vi "HOST_SviTockovi.vi"() -> ()   [LabVIEW 2014]
uses:
  <vilib>/rvi/interface/nirviOpenFPGA/nirviOpenFPGA.xnode
  <vilib>/rvi/interface/nirviReadWriteControl/nirviReadWriteControl.xnode
  <vilib>/rvi/interface/nirviCloseFPGA/nirviCloseFPGA.xnode
  <vilib>/FPGAPlugInAG/Dynamic/niLvFpga_Close_Dynamic.vi
  NiFpgaLv.dll
  <vilib>/Utility/error.llb/Error Cluster From Error Code.vi
  <vilib>/rvi/interface/Simulation/niFpgaSimulationCallBeginRW.vi
  <vilib>/rvi/errors/niLvFpgaAdjustHostInterfaceError.vi
  FPGA Bitfiles/UpravljanjeSaSvi_FPGATarget_Untitled2_yLwRjzwkvq8.lvbitx
  Untitled 2.vi
  <vilib>/FPGAPlugInAG/sbRIO-9636/niLvFpga_Open_sbRIO-9636.vi
  <vilib>/rvi/interface/common/dynamic/niFpgaDynamicAddResources.vi
panel:
  in  "stop":bool
  in  "naprijed":bool
  in  "dir 4":bool
  in  "dir 3":bool
  in  "dir 2":bool
  in  "dir 1":bool
  in  "rezolucija koraka":i32(listbox)
  in  "step":sgl(knob) scale=0.0..300.0
  in  "pokreni":bool
  in  "ulijevo":bool
  in  "udesno":bool
  in  "nazad":bool
  in  "rotacija udesno":bool
  in  "rotacija ulijevo":bool
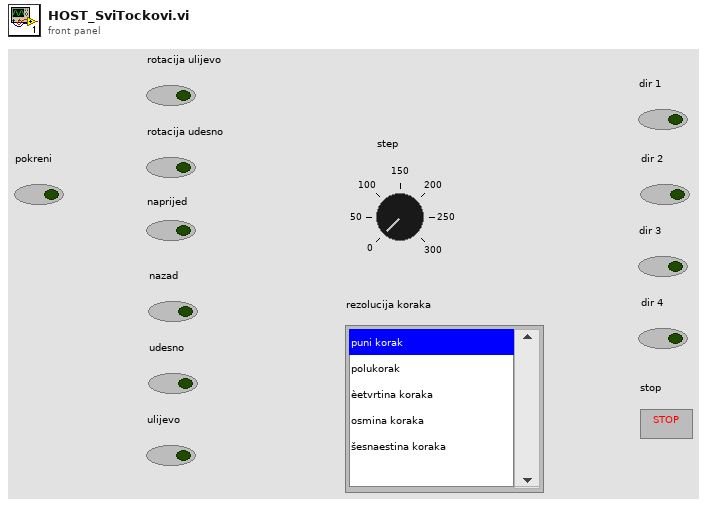
[diagram p1: front panel]
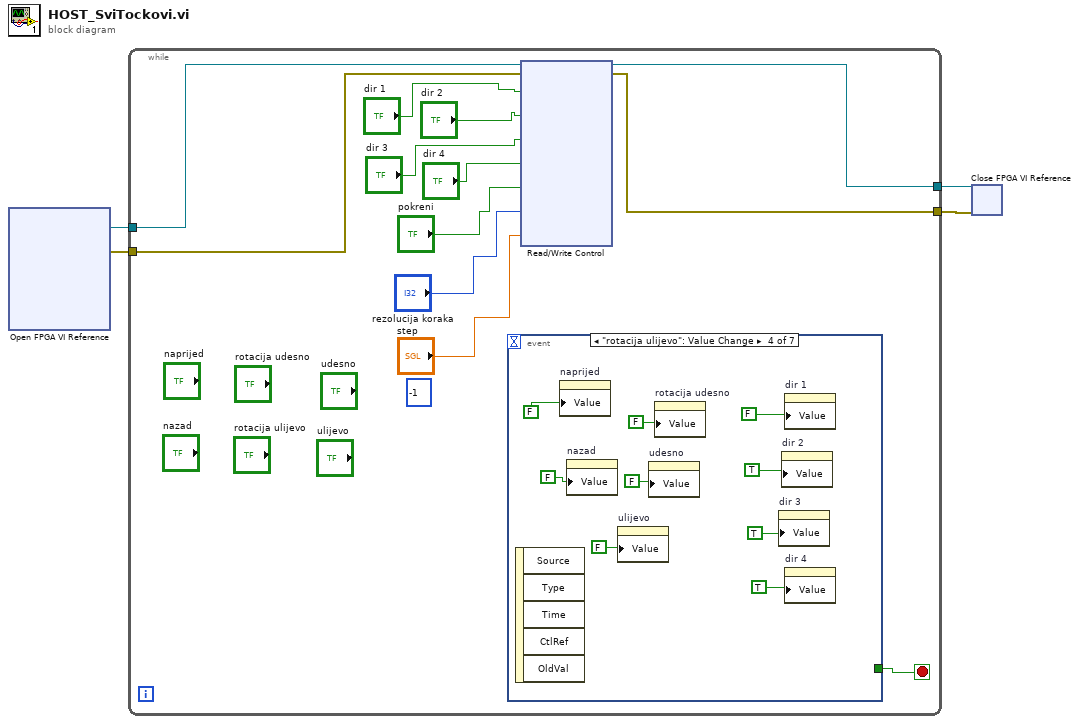
[diagram p0: block diagram]
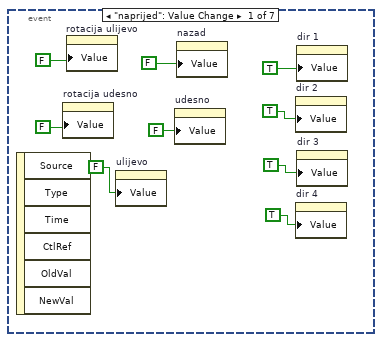
[diagram p2: hidden frame]
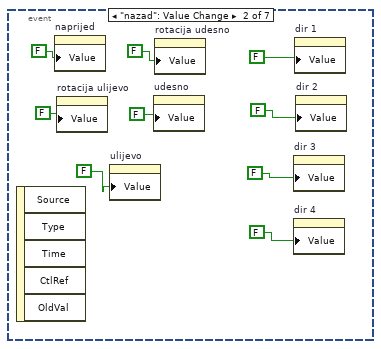
[diagram p3: hidden frame]
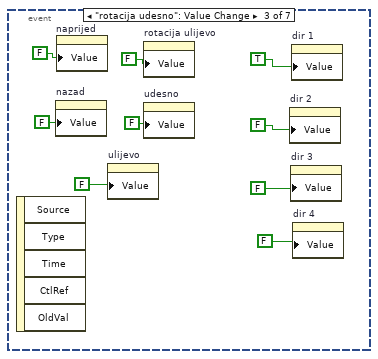
[diagram p4: hidden frame]
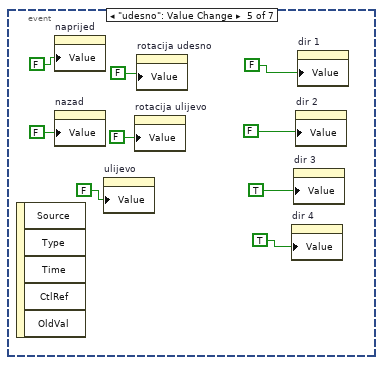
[diagram p5: hidden frame]
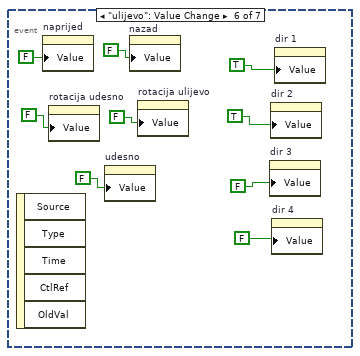
[diagram p6: hidden frame]
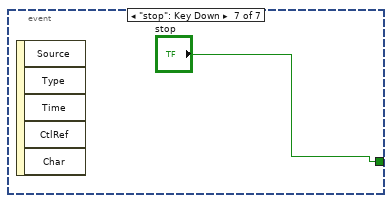
[diagram p7: hidden frame]
diagram:
  n1 = xnode "Open FPGA VI Reference"() -> ("FPGA VI Reference Out"=w3:refnum<k20>, "error out"=w4:errorcluster)  [unwired: 2 in]
  n2 = while {
    tunnel: w4 -> [w15]
    tunnel: w3 -> [w16]
    tunnel: [w14] -> w2
    tunnel: [w13] -> w1
    stop <- w5 stop-if-true
    (unwired) -1
    n3 = event shown="[3] \"rotacija ulijevo\": Value Change" {
      selector: _ -> [_ _ _ _ _ _ _]
      dyn-events: _ -> [_ _ _ _ _ _ _]
      timeout: _ -> [_ _ _ _ _ _ _]
      tunnel: [_ _ _ _ _ _ "stop"] -> w5
      event "naprijed": Value Change {
        n4 = event-data() -> ()  [unwired: 1 in, 6 out]
        n5 = property on="rotacija udesno" class="Bool (strict)"("Value"=FALSE) -> ()  [unwired: 2 in, 2 out]
        n6 = property on="rotacija ulijevo" class="Bool (strict)"("Value"=FALSE) -> ()  [unwired: 2 in, 2 out]
        n7 = property on="ulijevo" class="Bool (strict)"("Value"=FALSE) -> ()  [unwired: 2 in, 2 out]
        n8 = property on="udesno" class="Bool (strict)"("Value"=FALSE) -> ()  [unwired: 2 in, 2 out]
        n9 = property on="nazad" class="Bool (strict)"("Value"=FALSE) -> ()  [unwired: 2 in, 2 out]
        n10 = property on="dir 2" class="Bool (strict)"("Value"=TRUE) -> ()  [unwired: 2 in, 2 out]
        n11 = property on="dir 4" class="Bool (strict)"("Value"=TRUE) -> ()  [unwired: 2 in, 2 out]
        n12 = property on="dir 1" class="Bool (strict)"("Value"=TRUE) -> ()  [unwired: 2 in, 2 out]
        n13 = property on="dir 3" class="Bool (strict)"("Value"=TRUE) -> ()  [unwired: 2 in, 2 out]
      }
      event "nazad": Value Change {
        n14 = event-data() -> ()  [unwired: 1 in, 5 out]
        n15 = property on="naprijed" class="Bool (strict)"("Value"=FALSE) -> ()  [unwired: 2 in, 2 out]
        n16 = property on="rotacija ulijevo" class="Bool (strict)"("Value"=FALSE) -> ()  [unwired: 2 in, 2 out]
        n17 = property on="ulijevo" class="Bool (strict)"("Value"=FALSE) -> ()  [unwired: 2 in, 2 out]
        n18 = property on="udesno" class="Bool (strict)"("Value"=FALSE) -> ()  [unwired: 2 in, 2 out]
        n19 = property on="rotacija udesno" class="Bool (strict)"("Value"=FALSE) -> ()  [unwired: 2 in, 2 out]
        n20 = property on="dir 3" class="Bool (strict)"("Value"=FALSE) -> ()  [unwired: 2 in, 2 out]
        n21 = property on="dir 4" class="Bool (strict)"("Value"=FALSE) -> ()  [unwired: 2 in, 2 out]
        n22 = property on="dir 1" class="Bool (strict)"("Value"=FALSE) -> ()  [unwired: 2 in, 2 out]
        n23 = property on="dir 2" class="Bool (strict)"("Value"=FALSE) -> ()  [unwired: 2 in, 2 out]
      }
      event "rotacija udesno": Value Change {
        n24 = event-data() -> ()  [unwired: 1 in, 5 out]
        n25 = property on="nazad" class="Bool (strict)"("Value"=FALSE) -> ()  [unwired: 2 in, 2 out]
        n26 = property on="naprijed" class="Bool (strict)"("Value"=FALSE) -> ()  [unwired: 2 in, 2 out]
        n27 = property on="ulijevo" class="Bool (strict)"("Value"=FALSE) -> ()  [unwired: 2 in, 2 out]
        n28 = property on="rotacija ulijevo" class="Bool (strict)"("Value"=FALSE) -> ()  [unwired: 2 in, 2 out]
        n29 = property on="udesno" class="Bool (strict)"("Value"=FALSE) -> ()  [unwired: 2 in, 2 out]
        n30 = property on="dir 2" class="Bool (strict)"("Value"=FALSE) -> ()  [unwired: 2 in, 2 out]
        n31 = property on="dir 3" class="Bool (strict)"("Value"=FALSE) -> ()  [unwired: 2 in, 2 out]
        n32 = property on="dir 1" class="Bool (strict)"("Value"=TRUE) -> ()  [unwired: 2 in, 2 out]
        n33 = property on="dir 4" class="Bool (strict)"("Value"=FALSE) -> ()  [unwired: 2 in, 2 out]
      }
      event "rotacija ulijevo": Value Change {
        n34 = event-data() -> ()  [unwired: 1 in, 5 out]
        n35 = property on="naprijed" class="Bool (strict)"("Value"=FALSE) -> ()  [unwired: 2 in, 2 out]
        n36 = property on="nazad" class="Bool (strict)"("Value"=FALSE) -> ()  [unwired: 2 in, 2 out]
        n37 = property on="ulijevo" class="Bool (strict)"("Value"=FALSE) -> ()  [unwired: 2 in, 2 out]
        n38 = property on="udesno" class="Bool (strict)"("Value"=FALSE) -> ()  [unwired: 2 in, 2 out]
        n39 = property on="rotacija udesno" class="Bool (strict)"("Value"=FALSE) -> ()  [unwired: 2 in, 2 out]
        n40 = property on="dir 3" class="Bool (strict)"("Value"=TRUE) -> ()  [unwired: 2 in, 2 out]
        n41 = property on="dir 2" class="Bool (strict)"("Value"=TRUE) -> ()  [unwired: 2 in, 2 out]
        n42 = property on="dir 1" class="Bool (strict)"("Value"=FALSE) -> ()  [unwired: 2 in, 2 out]
        n43 = property on="dir 4" class="Bool (strict)"("Value"=TRUE) -> ()  [unwired: 2 in, 2 out]
      }
      event "udesno": Value Change {
        n44 = event-data() -> ()  [unwired: 1 in, 5 out]
        n45 = property on="naprijed" class="Bool (strict)"("Value"=FALSE) -> ()  [unwired: 2 in, 2 out]
        n46 = property on="nazad" class="Bool (strict)"("Value"=FALSE) -> ()  [unwired: 2 in, 2 out]
        n47 = property on="ulijevo" class="Bool (strict)"("Value"=FALSE) -> ()  [unwired: 2 in, 2 out]
        n48 = property on="rotacija ulijevo" class="Bool (strict)"("Value"=FALSE) -> ()  [unwired: 2 in, 2 out]
        n49 = property on="rotacija udesno" class="Bool (strict)"("Value"=FALSE) -> ()  [unwired: 2 in, 2 out]
        n50 = property on="dir 4" class="Bool (strict)"("Value"=TRUE) -> ()  [unwired: 2 in, 2 out]
        n51 = property on="dir 3" class="Bool (strict)"("Value"=TRUE) -> ()  [unwired: 2 in, 2 out]
        n52 = property on="dir 2" class="Bool (strict)"("Value"=FALSE) -> ()  [unwired: 2 in, 2 out]
        n53 = property on="dir 1" class="Bool (strict)"("Value"=FALSE) -> ()  [unwired: 2 in, 2 out]
      }
      event "ulijevo": Value Change {
        n54 = event-data() -> ()  [unwired: 1 in, 5 out]
        n55 = property on="naprijed" class="Bool (strict)"("Value"=FALSE) -> ()  [unwired: 2 in, 2 out]
        n56 = property on="rotacija udesno" class="Bool (strict)"("Value"=FALSE) -> ()  [unwired: 2 in, 2 out]
        n57 = property on="udesno" class="Bool (strict)"("Value"=FALSE) -> ()  [unwired: 2 in, 2 out]
        n58 = property on="nazad" class="Bool (strict)"("Value"=FALSE) -> ()  [unwired: 2 in, 2 out]
        n59 = property on="rotacija ulijevo" class="Bool (strict)"("Value"=FALSE) -> ()  [unwired: 2 in, 2 out]
        n60 = property on="dir 3" class="Bool (strict)"("Value"=FALSE) -> ()  [unwired: 2 in, 2 out]
        n61 = property on="dir 2" class="Bool (strict)"("Value"=TRUE) -> ()  [unwired: 2 in, 2 out]
        n62 = property on="dir 4" class="Bool (strict)"("Value"=FALSE) -> ()  [unwired: 2 in, 2 out]
        n63 = property on="dir 1" class="Bool (strict)"("Value"=TRUE) -> ()  [unwired: 2 in, 2 out]
      }
      event "stop": Key Down {
        n64 = event-data() -> ()  [unwired: 1 in, 5 out]
      }
    }
    n65 = xnode "Read/Write Control"("FPGA VI Reference In"=w16, "error in"=w15, "dir 1"="dir 1", "dir 2"="dir 2", "dir 3"="dir 3", "dir 4"="dir 4", "pokreni"="pokreni", "rezolucija"="rezolucija koraka", "step"="step") -> ("FPGA VI Reference Out"=w14:refnum<k20>, "error out"=w13:errorcluster)
  }
  n66 = xnode "Close FPGA VI Reference"("FPGA VI Reference In"=w2, "error in"=w1) -> ()  [unwired: 1 out]
